vi "CODMn核查数据输出格式 (子VI).vi"(11 "CODMn":string[](array[string])) -> (3 "字符串":string)   [LabVIEW 2016]
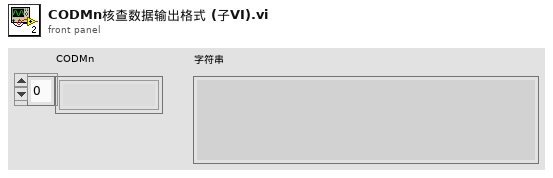
[diagram p1: front panel]
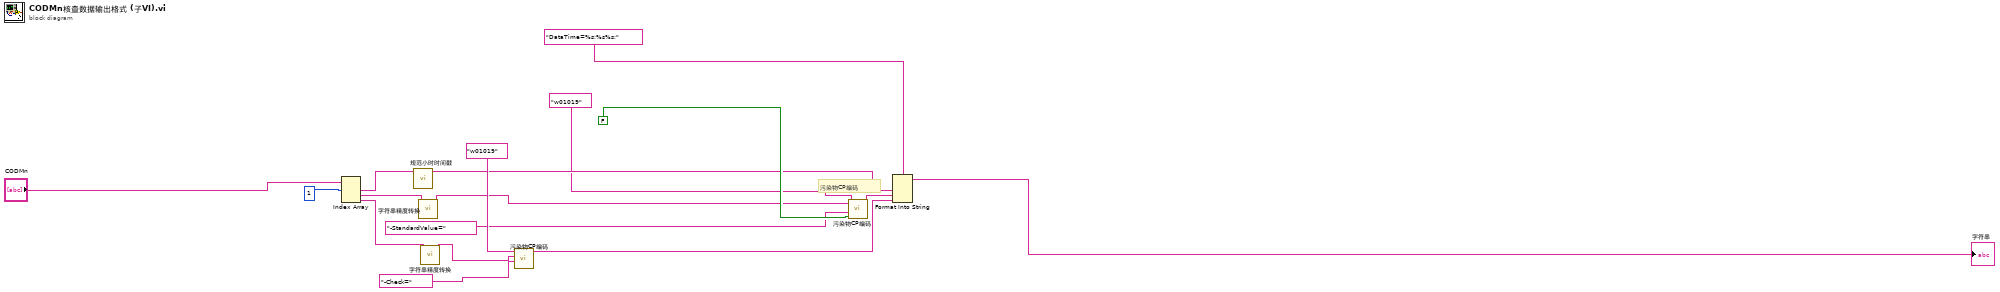
[diagram p0: block diagram]
diagram:
  # "污染物CP编码"
  n1 = Index Array(array="CODMn", index #1=1 ("索引")) -> (element #1=w4:string, element #2=w5:string, element #3=w12:string)  [unwired: 2 in]
  n2 = call "规范小时时间戳.vi"("字符串"=w4) -> ("result string"=w9:string)  [unwired: 10 in]
  n3 = call "字符串精度转换.vi"("输入字符串"=w5) -> ("输出字符串"=w6:string)  [unwired: 10 in]
  n4 = call "字符串精度转换.vi"("输入字符串"=w12) -> ("输出字符串"=w16:string)  [unwired: 10 in]
  n5 = call "污染物CP编码.vi"("数据类型"="-Check=", "污染物浓度"=w16, "污染物编码"="w01019") -> ("编码输出"=w13:string)  [unwired: 8 in]
  n6 = call "污染物CP编码.vi"("字段结束"=FALSE, "数据类型"="-StandardValue=", "污染物浓度"=w6, "污染物编码"="w01019") -> ("编码输出"=w8:string)  [unwired: 7 in]
  n7 = Format Into String(format string="DataTime=%s;%s%s;" ("格式字符串"), w9, w8, w13) -> (resulting string=→"字符串":string)  [unwired: 2 in, 1 out]
